vi "Buzz20_Main.vi"() -> ()   [LabVIEW 2015]
uses:
  <vilib>/Platform/TimedLoop/XDataNode/XDataNode.xnode
  <vilib>/Platform/TimedLoop/XDataNode/timing_clust.ctl
  <vilib>/Platform/TimedLoop/XDataNode/XDNodeRunTimeDep.lvlib
  <vilib>/Platform/TimedLoop/XDataNode/wakeup.ctl
  <vilib>/Platform/TimedLoop/XDataNode/nitl_modes.ctl
  <vilib>/NI_Real-Time Target Support.lvlib
  Gensubs/Bert_or_Ernie.vi
  Typedefs/JoysticksGlobal.vi
  Typedefs/GamepadData.ctl
  Typedefs/ActuatorInputs.ctl
  Typedefs/SensorInputData.ctl
  <vilib>/Utility/RT CPU Load.ctl
  Typedefs/Arm States.ctl
  Typedefs/HMI_to_Control.ctl
  Typedefs/IntakeWheelSenseOrManual.ctl
  Typedefs/ClawStates.ctl
panel:
  out "Error":errorcluster
  in  "On Bert?":bool=TRUE
  out "HMI to ControlOut":T1
  in  "HMI to Control":T1
  out "CPU loads":T5[](array[typedef]) {"ISR (%)" format="%#.2f"; "Idle (%)" format="%#.2f"; "Background (%)" format="%#.2f"; "Normal (%)" format="%#.2f"; "Above Normal (%)" format="%#.2f"; "High (%)" format="%#.2g"; "Timed Structures (%)" format="%#.2g"; "Time Critical (%)" format="%#.2g"; "Total (%)" format="%#.2g"}
  out "SensorInputDataOut":T6
  in  "SensorInputData":T6
  out "OpenSuccesfull":bool
  in  "ActuatorInputs":T7
  in  "GamepadData":T8
  out "ActuatorInputsOut":T7
  out "GamepadDataOut":T8
  out "Finished Late? [i-1]":bool
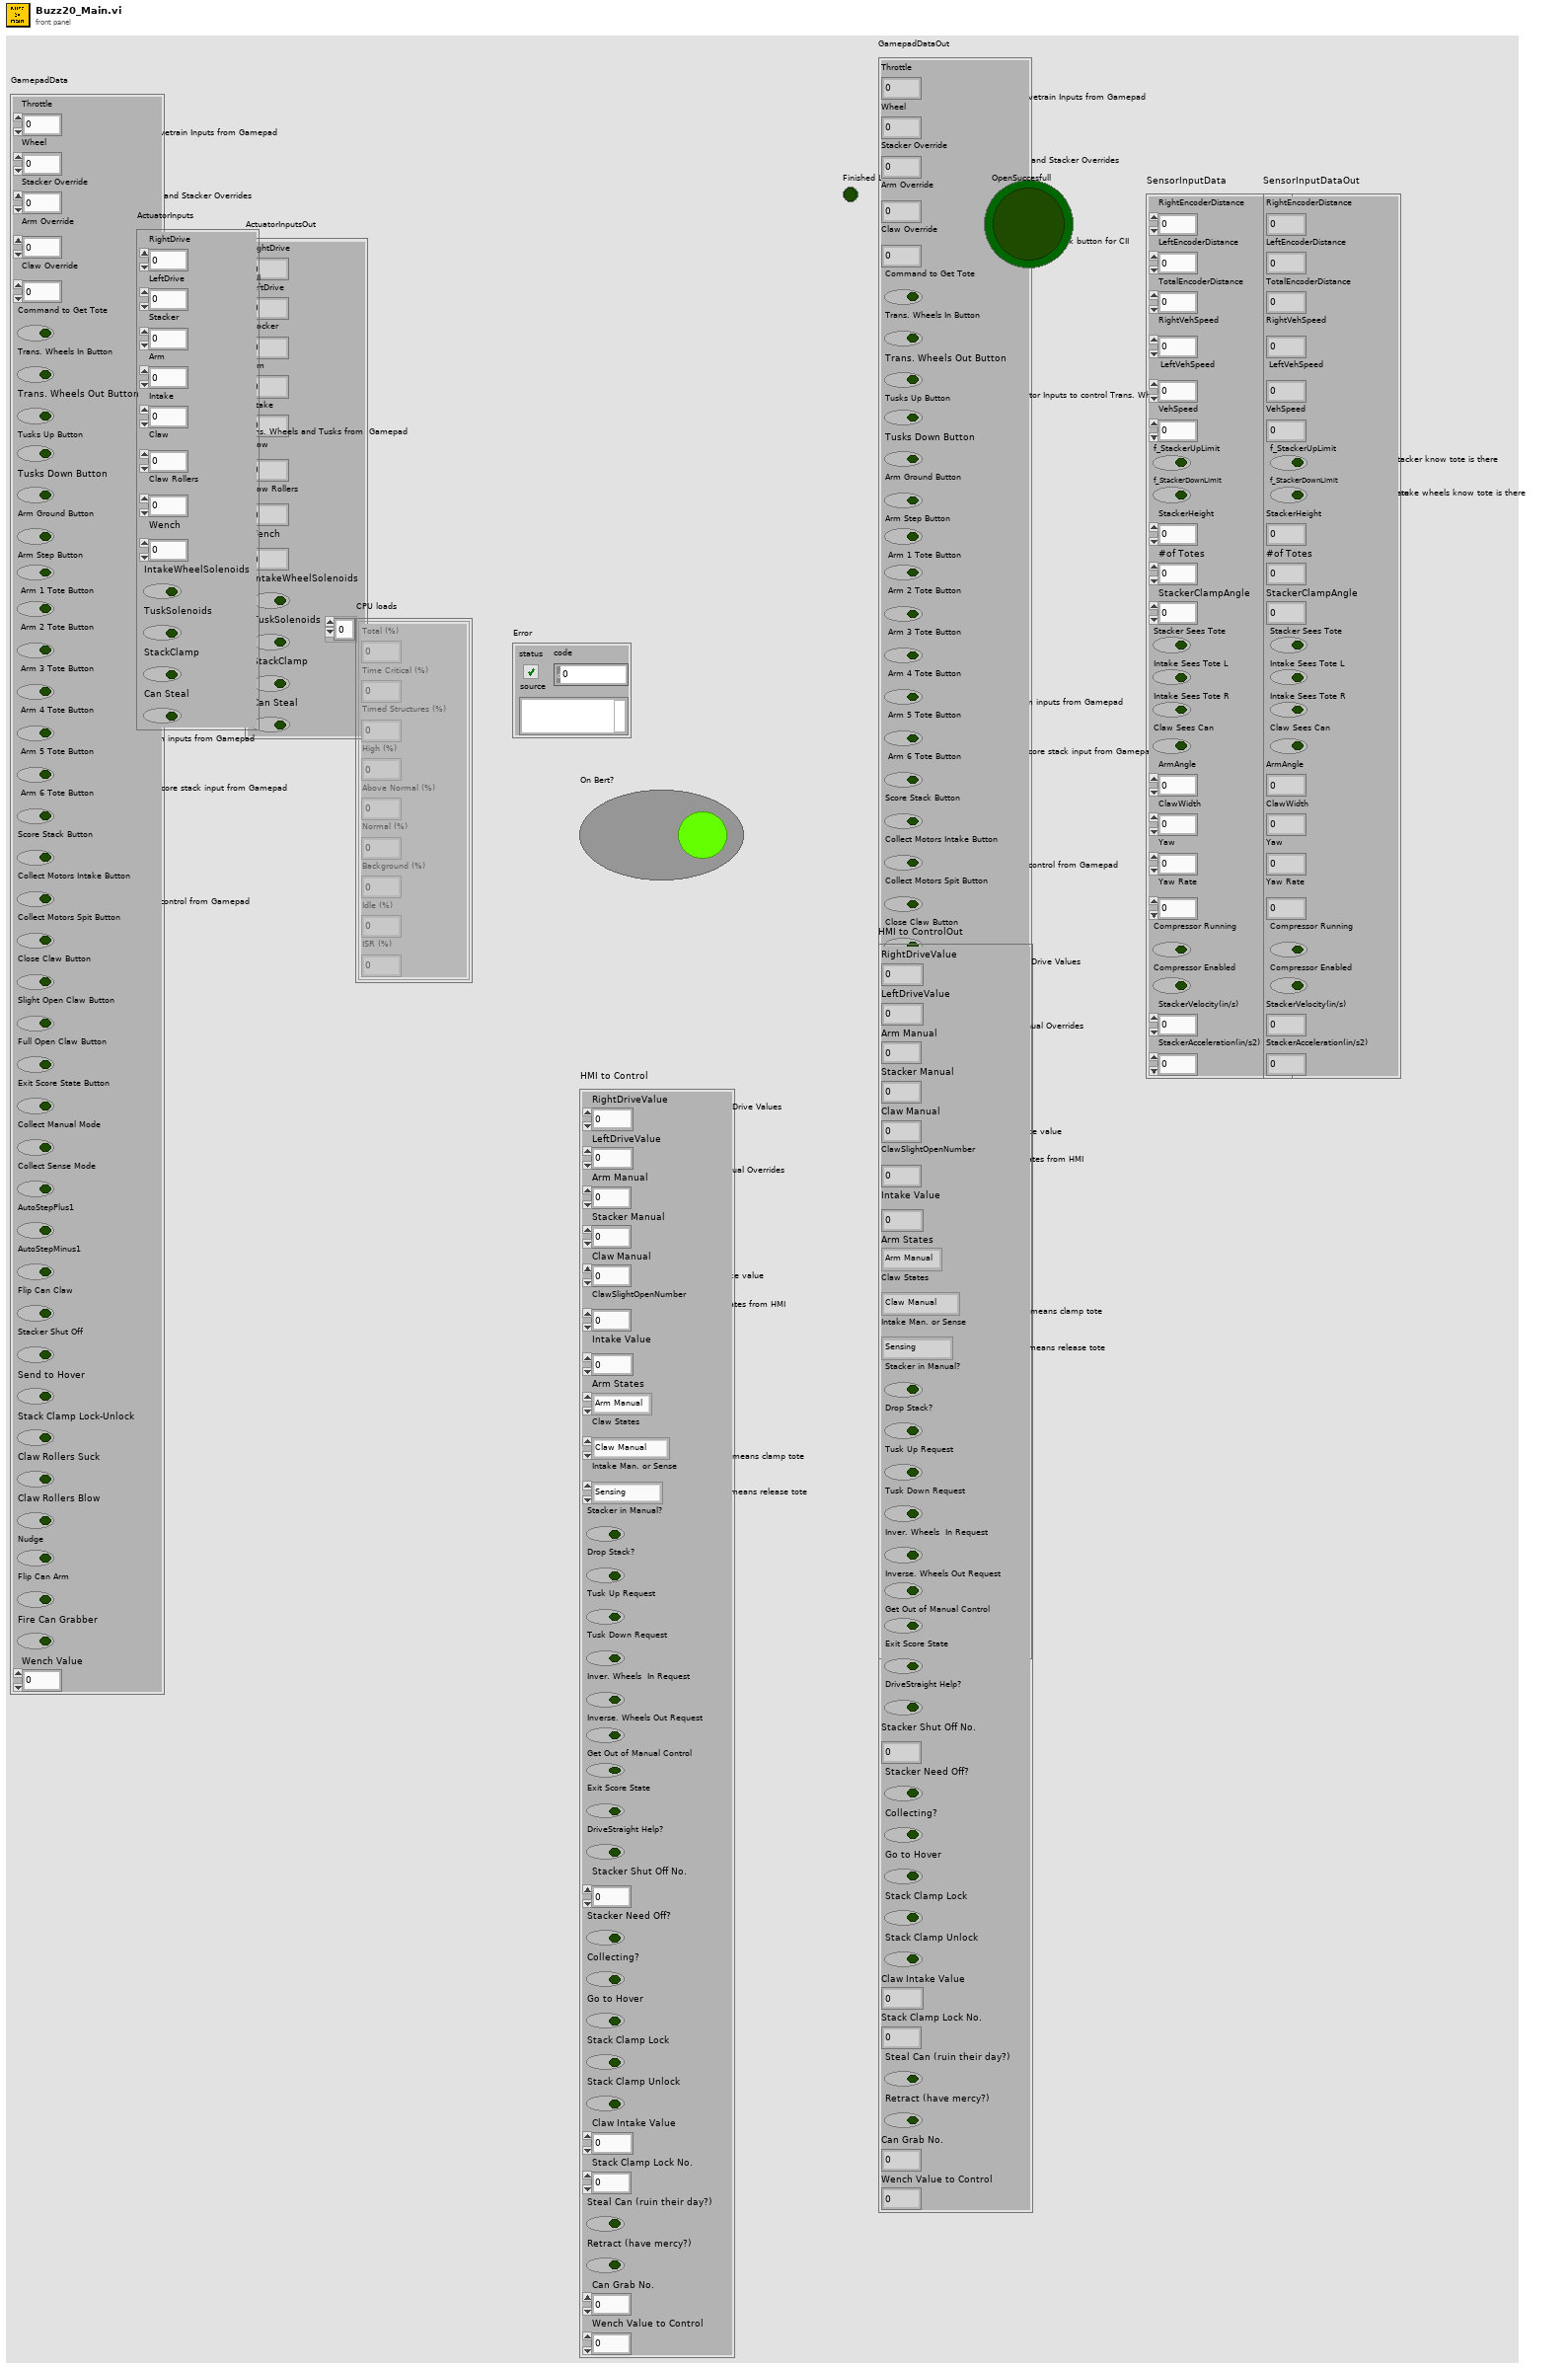
[diagram p1: front panel]
types:
  T1 = typedef "HMI_to_Control.ctl" = cluster{"RightDriveValue":dbl, "LeftDriveValue":dbl, "Arm Manual ":dbl, "Stacker Manual ":dbl, "Claw Manual ":dbl, "ClawSlightOpenNumber":i8, "Intake Value ":sgl, "Arm States":T2, "Claw States":T3, "Intake Man. or Sense":T4, "Stacker in Manual?":bool, "Drop Stack? ":bool, "Tusk Up Request":bool, "Tusk Down Request":bool, "Inver. Wheels  In Request":bool, "Inverse. Wheels Out Request ":bool, "Get Out of Manual Control":bool, "Exit Score State":bool, "DriveStraight Help?":bool, "Stacker Shut Off No.":i8, "Stacker Need Off?":bool, "Collecting?":bool, "Go to Hover":bool, "Stack Clamp Lock ":bool, "Stack Clamp Unlock ":bool, "Claw Intake Value ":sgl, "Stack Clamp Lock No. ":i8, "Steal Can (ruin their day?)":bool, "Retract (have mercy?)":bool, "Can Grab No. ":i8, "Wench Value to Control ":dbl}
  T2 = typedef "Arm States.ctl" = enum16{"Arm Manual ", "Ground", "Step", "1 Tote", "2 Tote", "3 Tote", "4 Tote", "5 Tote", "6 Tote", "Flip Can Arm", "Grab Can in auto", "Nudge"}
  T3 = typedef "ClawStates.ctl" = enum16{"Claw Manual ", "Claw Open", "Claw Closed", "Claw Slight Open", "Flip Can"}
  T4 = typedef "IntakeWheelSenseOrManual.ctl" = enum16{"Sensing", "Manual "}
  T5 = typedef "NI_Real-Time Target Support.lvlib/RT CPU Load.ctl" = cluster{"Total (%)":dbl, "Time Critical (%)":dbl, "Timed Structures (%)":dbl, "High (%)":dbl, "Above Normal (%)":dbl, "Normal (%)":dbl, "Background (%)":dbl, "Idle (%)":dbl, "ISR (%)":dbl}
  T6 = typedef "SensorInputData.ctl" = cluster{"RightEncoderDistance":dbl, "LeftEncoderDistance":dbl, "TotalEncoderDistance":dbl, "RightVehSpeed":dbl, "LeftVehSpeed":dbl, "VehSpeed":dbl, "f_StackerUpLimit":bool, "f_StackerDownLimit":bool, "StackerHeight":dbl, "#of Totes":u8, "StackerClampAngle":dbl, "Stacker Sees Tote":bool, "Intake Sees Tote L":bool, "Intake Sees Tote R":bool, "Claw Sees Can":bool, "ArmAngle":dbl, "ClawWidth":dbl, "Yaw":dbl, "Yaw Rate":dbl, "Compressor Running":bool, "Compressor Enabled":bool, "StackerVelocity(in/s)":dbl, "StackerAcceleration(in/s2)":dbl}
  T7 = typedef "ActuatorInputs.ctl" = cluster{"RightDrive":dbl, "LeftDrive":dbl, "Stacker":dbl, "Arm":dbl, "Intake":sgl, "Claw":dbl, "Claw Rollers":i8, "Wench":dbl, "IntakeWheelSolenoids":bool, "TuskSolenoids":bool, "StackClamp":bool, "Can Steal":bool}
  T8 = typedef "GamepadData.ctl" = cluster{"Throttle":dbl, "Wheel":dbl, "Stacker Override":dbl, "Arm Override ":dbl, "Claw Override":dbl, "Command to Get Tote":bool, "Trans. Wheels In Button":bool, "Trans. Wheels Out Button":bool, "Tusks Up Button":bool, "Tusks Down Button":bool, "Arm Ground Button":bool, "Arm Step Button":bool, " Arm 1 Tote Button":bool, " Arm 2 Tote Button":bool, " Arm 3 Tote Button ":bool, " Arm 4 Tote Button":bool, " Arm 5 Tote Button":bool, " Arm 6 Tote Button":bool, "Score Stack Button":bool, "Collect Motors Intake Button":bool, "Collect Motors Spit Button":bool, "Close Claw Button":bool, "Slight Open Claw Button":bool, "Full Open Claw Button ":bool, "Exit Score State Button":bool, "Collect Manual Mode ":bool, "Collect Sense Mode":bool, "AutoStepPlus1":bool, "AutoStepMinus1":bool, "Flip Can Claw":bool, "Stacker Shut Off":bool, "Send to Hover ":bool, "Stack Clamp Lock-Unlock ":bool, "Claw Rollers Suck ":bool, "Claw Rollers Blow ":bool, "Nudge":bool, "Flip Can Arm ":bool, "Fire Can Grabber":bool, "Wench Value":dbl}
  T9 = typedef "WPI_JoystickDevRef.ctl" = cluster{"Device":T10}
  T10 = typedef "WPI_JoystickDeviceEnum.ctl" = enum16{"USB 0", "USB 1", "USB 2", "USB 3", "USB 4", "USB 5"}
  T11 = typedef "WPI_PotentiometerDevRef.ctl" = cluster{"DevStatus":errorcluster, "Analog Channel":T12, "Invert Output":bool}
  T12 = typedef "FPGA_AIChannel.ctl" = enum8{"AI 0", "AI 1", "AI 2", "AI 3", "AI MXP 0", "AI MXP 1", "AI MXP 2", "AI MXP 3", "Invalid"}
  T13 = typedef "WPI_EncoderDevRef.ctl" = cluster{"DevStatus":errorcluster, "EncoderIndex":T14, "CounterIndex":T15, "DistancePerCount":dbl, "Decoding Type":T16}
  T14 = typedef "FPGA_EncoderIdx.ctl" = enum8{"Enc 0", "Enc 1", "Enc 2", "Enc 3", "Enc 4", "Enc 5", "Enc 6", "Enc 7", "Invalid"}
  T15 = typedef "FPGA_CounterCtrSystemIndex.ctl" = enum8{"Ctr 0", "Ctr 1", "Ctr 2", "Ctr 3", "Ctr 4", "Ctr 5", "Ctr 6", "Ctr 7", "Invalid"}
  T16 = typedef "WPI_EncoderType.ctl" = enum16{"1x", "2x", "4x"}
  T17 = typedef "WPI_SwitchDevRef.ctl" = cluster{"DevStatus":errorcluster, "DIO Channel":T18, "CntIndex":T15, "Normally Closed":bool}
  T18 = typedef "FPGA_DIOChannel.ctl" = enum8{"DIO 0", "DIO 1", "DIO 2", "DIO 3", "DIO 4", "DIO 5", "DIO 6", "DIO 7", "DIO 8", "DIO 9", "DIO MXP 0", "DIO MXP 1", "DIO MXP 2", "DIO MXP 3", "DIO MXP 4", "DIO MXP 5", "DIO MXP 6", "DIO MXP 7", "DIO MXP 8", "DIO MXP 9", "DIO MXP 10", "DIO MXP 11", "DIO MXP 12", "DIO MXP 13", "DIO MXP 14", "DIO MXP 15", "Invalid"}
  T19 = typedef "WPI_GyroDevRef.ctl" = cluster{"DevStatus":errorcluster, "Analog Channel":T12, "Offset":dbl, "Gain (VoltsPerDegree/Second)":dbl, "Gyro Type":enum16{"Analog", "XRS450"}, "Handle":i32, "SPI Bus":T20, "Device Found":bool, "Sample Rate":dbl, "Calibrate On Open":bool}
  T20 = typedef "spi_bus.ctl" = enum16{"SPI On-Board, CS0", "SPI On-Board, CS1", "SPI On-Board, CS2", "SPI On-Board, CS3", "SPI MXP", "Invalid"}
  T21 = typedef "WPI_CompressorDevRef.ctl" = cluster{"DevStatus":errorcluster, "Pneumatics Control Module":u8}
  T22 = cluster{T9[], cluster{T11[], T13[], T17[], "GyroDevRef":T19, "CompressorDevRef":T21}}
  T23 = typedef "WPI_MotorControlDeviceRef.ctl" = cluster{"DeviceStatus":errorcluster, "Type":T24, "PWM":cluster{"PWM Channel":T25, "DeadBand":T26}, "CAN":cluster{"Device Number":u8, "Control Mode":T27, "Semaphore":T28, "Max Vout":dbl, "TalonSRX Control Mode":T29}, "Invert":bool}
  T24 = typedef "WPI_MotorControlType.ctl" = enum16{"PWM", "CAN", "CANTalonSRX"}
  T25 = typedef "FPGA_DIOPWMChannel.ctl" = enum8{"PWM 0", "PWM 1", "PWM 2", "PWM 3", "PWM 4", "PWM 5", "PWM 6", "PWM 7", "PWM 8", "PWM 9", "PWM MXP 0", "PWM MXP 1", "PWM MXP 2", "PWM MXP 3", "PWM MXP 4", "PWM MXP 5", "PWM MXP 6", "PWM MXP 7", "PWM MXP 8", "PWM MXP 9", "Invalid"}
  T26 = typedef "WPI_PWMDeadband.ctl" = cluster{"Name":string, "maxPositivePwm":i32, "minPositivePwm":i32, "centerPwm":i32, "maxNegativePwm":i32, "minNegativePwm":i32, "angularRange":u16}
  T27 = typedef "WPI_CANJaguar_ControlMode.ctl" = enum8{"Percent VBus", "Current", "Speed", "Position", "Voltage"}
  T28 = typedef "Semaphore RefNum" = refnum<k1>
  T29 = typedef "WPI_CANTalonSRX_APIControlMode.ctl" = enum8{"Percent VBus", "Speed", "Position", "Slave", "Unchanged / Invalid", "Voltage Compensation", "Current", "Motion Profile"}
  T30 = typedef "WPI_SolenoidDevRef.ctl" = cluster{"DevStatus":errorcluster, "Pneumatics Control Module":u8, "Forward Solenoid Channel":T31, "Reverse Solenoid Channel":T31}
  T31 = typedef "WPI_SolenoidChannel.ctl" = enum8{"Solenoid 0", "Solenoid 1", "Solenoid 2", "Solenoid 3", "Solenoid 4", "Solenoid 5", "Solenoid 6", "Solenoid 7", "Invalid"}
  T32 = typedef "WPI_SPIDevRef.ctl" = cluster{"DevStatus":errorcluster, "Handle":i32, "SPI Bus":T20}
  T33 = typedef "XDNodeRunTimeDep.lvlib/timing_clust.ctl" = cluster{"Expected End [f-1]":u64, "Actual End [f-1]":u64, "Finished Late? [f-1]":bool, "Expected End [i-1]":u64, "Actual End [i-1]":u64, "Finished Late? [i-1]":bool, "Expected Start [i]":u64, "Actual Start [i]":u64, "Expected Start [f]":u64, "Actual Start [f]":u64, "Source Name":string, "Structure Name":string, "Period":i64, "Deadline":i64, "Offset":i64, "Start":i64, "Priority":i32, "Timeout":i32, "Mode":T34, "Wakeup Reason":T35, "Error":errorcluster, "Source Type":string, "Secondary Source Type":string, "Global End Time":u64, "Global Start Time":u64, "Frame Duration":u64, "Iteration Duration":u64, "Assigned CPU":i32, "I/O Scan Engine Mode":u32}
  T34 = typedef "XDNodeRunTimeDep.lvlib/nitl_modes.ctl" = enum32{"No Change", "Process missed periods, maintain original phase", "Discard missed periods, maintain original phase", "Process missed periods, ignore original phase", "Discard missed periods, ignore original phase"}
  T35 = typedef "XDNodeRunTimeDep.lvlib/wakeup.ctl" = enum32{"Normal", "Aborted", "Asynchronous wakeup", "Timing source error", "Timed loop error", "Timeout"}
  T36 = cluster{"Axes":dbl[], "Buttons":bool[], "POVs":i16[]}
  T37 = cluster{cluster{"Axes":dbl[], "Buttons":bool[], "POVs":i16[]}, cluster{"Axes":dbl[], "Buttons":bool[], "POVs":i16[]}, cluster{"Axes":dbl[], "Buttons":bool[], "POVs":i16[]}}
  T38 = typedef "NetComm_ControlWord.ctl" = cluster{"Enabled":bool, "Autonomous":bool, "Test":bool, "E-Stop":bool, "FMS Attached":bool, "DS Attached":bool}
  T39 = typedef "WPI_DriverStationRobotMode2.ctl" = enum16{"Autonomous Disabled", "Autonomous Enabled", "Teleop Disabled", "Teleop Enabled", "Disconnected", "Finish", "Test Disabled", "Test Enabled", "Emergency Stopped"}
  T40 = typedef "StackerToDashboardData.ctl" = cluster{"# of Totes Out":i32, "Stacker State to Index":T41, "Stacker Off?":bool, "Stack Clamp Locked?":bool}
  T41 = typedef "StackerStates.ctl" = enum16{"Manual ", "Hold", "Hold5", "Hold6", "GetTote", "DropStack", "Hover", "Hover5", "Wait for Up", "DecideHold", "DownTimerPeriod", "Prep Intake for Drop", "Check Arm before 5", "Make Arm ready for 5", "Check Arm before 6", "Make Arm ready for 6", "Delay for 5", "Delay for 6"}
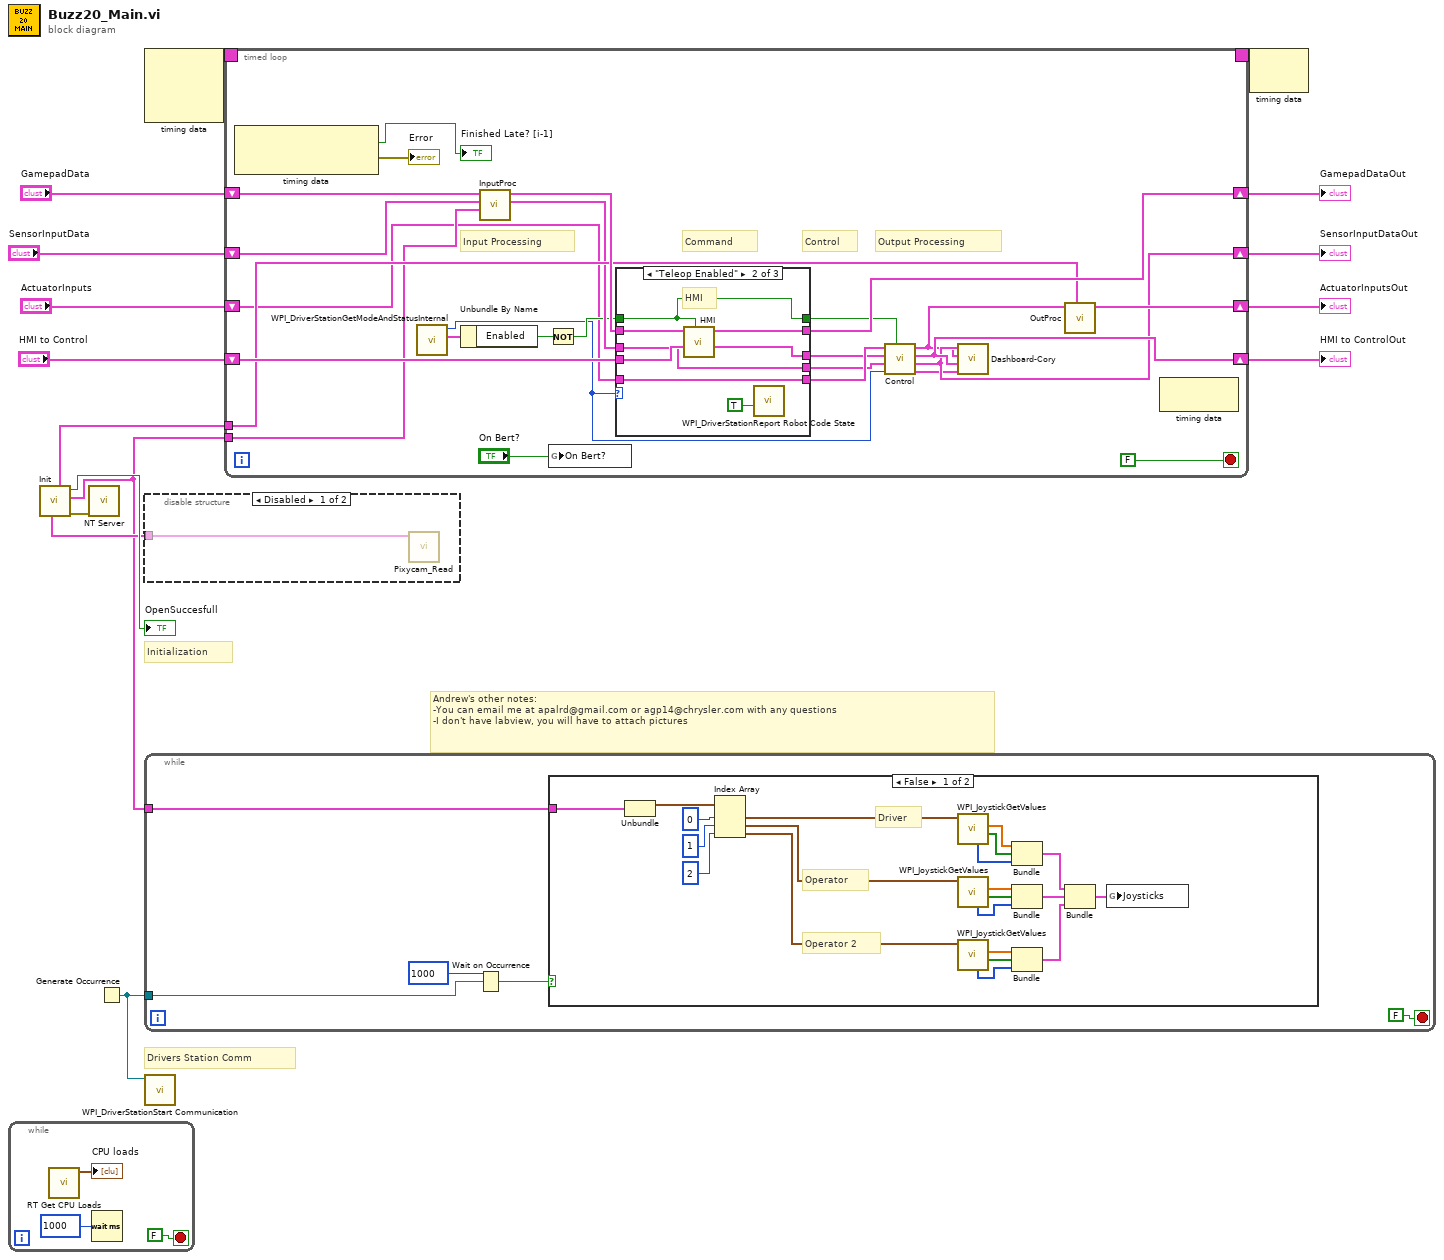
[diagram p0: block diagram]
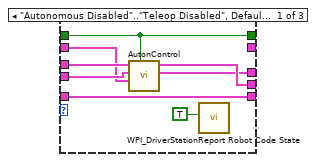
[diagram p4: hidden frame]
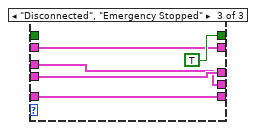
[diagram p5: hidden frame]
diagram:
  # "Drivers Station Comm"
  # "Andrew's other notes:\n-You can email me at apalrd@gmail.com or agp14@chrysler.com with any questions\n-I don't have labview, you will have to attach pictures"
  # "Initialization"
  n1 = while {
    stop <- FALSE stop-if-true
    n2 = call <vilib>:"RT Get CPU Loads.vi"() -> ("CPU loads"=→"CPU loads":T5[])  [unwired: 10 in, 1 out]
    n3 = Wait (ms)(milliseconds to wait=u32 1000) -> ()  [unwired: 1 out]
  }
  n4 = call "Init.vi"() -> ("error out"=w1:errorcluster, "output cluster"=w3:T22, "OpenSuccesfull"=→"OpenSuccesfull":bool, "Motor & Solonoid Cluster"=w7:cluster{T23[], T30[]}, "PixySPIDevRef"=w6:T32)  [unwired: 7 in]
  n5 = call <vilib>:"NT Server.vi"("error in (no error)"=w1) -> ()  [unwired: 11 in]
  n6 = Generate Occurrence() -> (w2:refnum<k4>)
  n7 = node-c288() -> (w16:T33)  [unwired: 3 in]
  n8 = disable-structure shown="Disabled" {
    disable-tunnel: w6 -> [w20 _]
    frame Disabled {
      n9 = call "Pixycam_Read.vi"("PixySPIDevRef"=w20) -> ()  [unwired: 11 in]
    }
    frame Enabled {
    }
  }
  n10 = while {
    tunnel: w3 -> [w21]
    tunnel: w2 -> [w24]
    stop <- FALSE stop-if-true
    n11 = Wait on Occurrence(2:w24, 3:1000 ("ms timeout (-1)")) -> (0:w23:bool)  [unwired: 1 in]
    n12 = case shown="False" w23 {
      tunnel: w21 -> [w40 _]
      frame False {
        # "Operator 2"
        # "Operator"
        # "Driver"
        n13 = Unbundle(w40) -> (w39:T9[])  [unwired: 1 out]
        n14 = Index Array(array=w39, index #1=0 ("index"), index #2=1 ("index"), index #3=2 ("index")) -> (element #1=w45:T9, element #2=w44:T9, element #3=w46:T9)
        n15 = call <vilib>:"WPI_JoystickGetValues.vi"("JoystickDevRef"=w45) -> ("Buttons"=w37:bool[], "Axes"=w38:dbl[], "POVs"=w36:i16[])  [unwired: 6 in, 2 out]
        n16 = call <vilib>:"WPI_JoystickGetValues.vi"("JoystickDevRef"=w44) -> ("Buttons"=w34:bool[], "Axes"=w35:dbl[], "POVs"=w33:i16[])  [unwired: 6 in, 2 out]
        n17 = call <vilib>:"WPI_JoystickGetValues.vi"("JoystickDevRef"=w46) -> ("Buttons"=w31:bool[], "Axes"=w32:dbl[], "POVs"=w30:i16[])  [unwired: 6 in, 2 out]
        n18 = Bundle("Axes"=w38, "Buttons"=w37, "POVs"=w36) -> (w29:T36)  [unwired: 1 in]
        n19 = Bundle("Axes"=w35, "Buttons"=w34, "POVs"=w33) -> (w28:T36)  [unwired: 1 in]
        n20 = Bundle("Axes"=w32, "Buttons"=w31, "POVs"=w30) -> (w27:T36)  [unwired: 1 in]
        n21 = Bundle(w29, w28, w27) -> (w26:T37)  [unwired: 1 in]
        n22 = global write "JoysticksGlobal.vi" "Joysticks"(w26) -> ()
      }
      frame True {
      }
    }
  }
  n23 = call <vilib>:"WPI_DriverStationStart Communication.vi"("occurrence"=w2) -> ()  [unwired: 1 in, 10 out]
  n24 = timed-loop {
    timing: w16 -> [_]
    timing-out: [_] -> w15
    shift-right: [w70] -> w14
    shift-left: "GamepadData" -> [w67]
    shift-right: [w63] -> w13
    shift-left: "ActuatorInputs" -> [w48]
    shift-right: [w62] -> w4
    shift-left: "HMI to Control" -> [w69]
    shift-right: [w61] -> w8
    shift-left: "SensorInputData" -> [w66]
    tunnel: w7 -> [w64]
    tunnel: w3 -> [w55]
    stop <- FALSE stop-if-true
    # "Output Processing"
    # "Control"
    # "Command"
    # "Input Processing"
    n25 = node-c288() -> (→"Finished Late? [i-1]":bool, →"Error":errorcluster)  [unwired: 1 in]
    n26 = call <vilib>:"WPI_DriverStationGetModeAndStatusInternal.vi"() -> ("Control Word"=w51:T38, "Robot Mode"=w47:T39)  [unwired: 10 in]
    n27 = Unbundle By Name(w51) -> ("Enabled"=w50:bool)
    n28 = call "InputProc.vi"("output cluster"=w55, "SensorInputData"=w66, "GamepadData"=w67) -> ("SensorInputDataOut"=w58:T6, "GamepadDataOut"=w65:T8)  [unwired: 5 in, 1 out]
    n29 = Not(x=w50) -> (.not. x?=w49:bool)
    n30 = global write "Bert_or_Ernie.vi" "On Bert?"("On Bert?") -> ()
    n31 = case shown="\"Teleop Enabled\"" w47 {
      tunnel: w65 -> [w73 w87 w92]
      tunnel: [_ w86 w92] -> w70
      tunnel: w48 -> [w79 w84 w91]
      tunnel: w69 -> [w77 w85 w90]
      tunnel: [w79 w84 w91] -> w68
      tunnel: w58 -> [w78 w83 w89]
      tunnel: [w76 w83 w89] -> w57
      tunnel: [w75 w82 w90] -> w56
      tunnel: [w74 w81 TRUE ("Disabled?")] -> w52
      tunnel: w49 -> [w74 w81 _]
      frame "Autonomous Disabled".."Teleop Disabled", Default {
        n32 = call "AutonControl.vi"("Disabled"=w74, "Gamepad Data"=w73, "HMI to Control"=w77, "SensorInputData"=w78) -> ("HMI to Control Out"=w75:T1, "SensorInputDataOut"=w76:T6)  [unwired: 5 in, 1 out]
        n33 = call <vilib>:"WPI_DriverStationReport Robot Code State.vi"("Autonomous"=TRUE) -> ()  [unwired: 10 in, 1 out]
      }
      frame "Teleop Enabled" {
        # "HMI"
        n34 = call "HMI.vi"("Disabled?"=w81, "HMI to Control"=w85, "GamepadData"=w87) -> ("HMI to Control Out"=w82:T1, "GamepadDataOut"=w86:T8)  [unwired: 5 in]
        n35 = call <vilib>:"WPI_DriverStationReport Robot Code State.vi"("TeleOp"=TRUE) -> ()  [unwired: 10 in, 1 out]
      }
      frame "Disconnected", "Emergency Stopped" {
      }
    }
    n36 = call "Control.vi"("Disabled"=w52, "RobotMode"=w47, "SensorInputData"=w57, "HMI to Control"=w56, "ActuatorInputs"=w68) -> ("Stacker to Dashboard Out"=w53:T40, "SensorInputDataOut"=w61:T6, "HMI to Control Out"=w62:T1, "ActuatorInputsOut"=w60:T7)  [unwired: 3 in]
    n37 = call "Dashboard-Cory.vi"("SensorInputData"=w61, "ActuatorInputs"=w60, "HMI to Control"=w62, "Stacker to Dashboard"=w53) -> ()  [unwired: 6 in]
    n38 = call "OutProc.vi"("Motor Cluster In"=w64, "ActuatorInputs"=w60) -> ("ActuatorInputsOut"=w63:T7)  [unwired: 9 in]
    n39 = node-c288() -> ()  [unwired: 1 in, 1 out]
  }
  "GamepadDataOut" <- w14
  "ActuatorInputsOut" <- w13
  "SensorInputDataOut" <- w8
  "HMI to ControlOut" <- w4
  n40 = node-c288(w15) -> ()  [unwired: 1 out]
